vi "midi_TicsToTime.vi"(8 "error in (no error)":errorcluster, 9 "ticks per qnote":u16, 10 "tempo":u32[][](array[numeric]), 11 "notes in":u32[][](array[numeric])) -> (0 "error out":errorcluster, 2 "duration (s)":dbl, 3 "notes out":dbl[][](array[numeric]))   [LabVIEW 2013]
doc: "Convert the start times and durations from \"tics\" to seconds."
uses:
  <vilib>/Analysis/NI_AALPro.lvlib
panel:
  # "midi_TicsToTime"
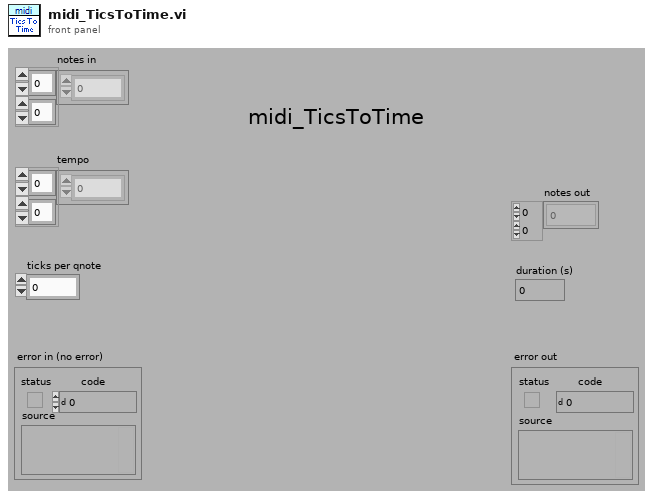
[diagram p1: front panel]
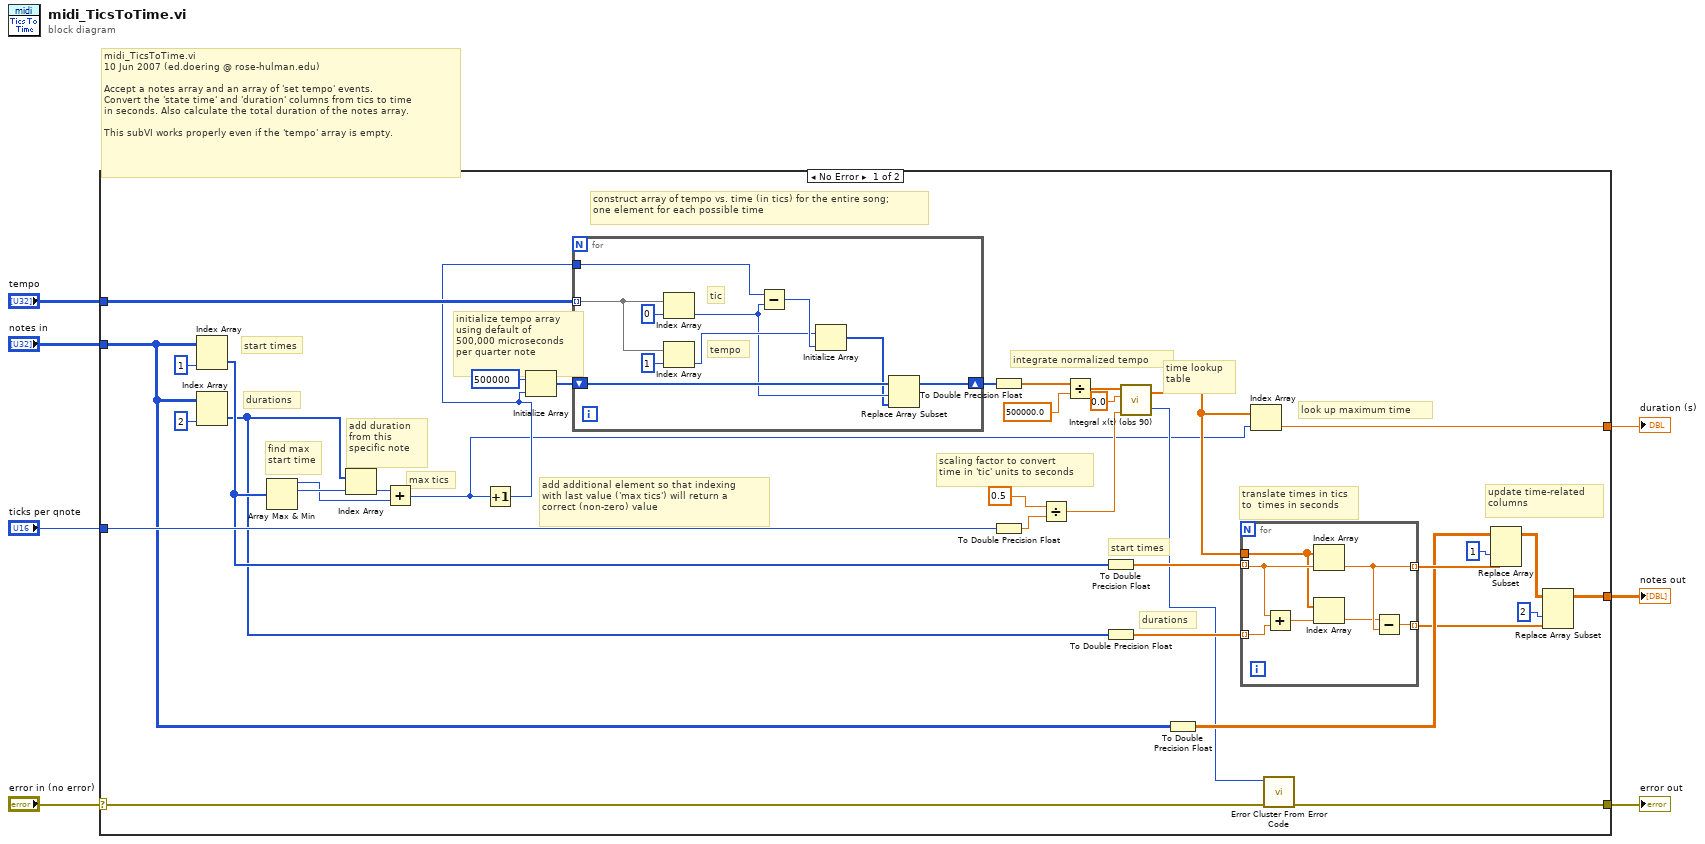
[diagram p0: block diagram]
diagram:
  # "midi_TicsToTime.vi\n10 Jun 2007 (ed.doering @ rose-hulman.edu)\n\nAccept a notes array and an array of 'set tempo' events.\nConvert the 'state time' and 'duration' columns from tics to time\nin seconds. Also calculate the total duration of the notes array.\n\nThis subVI works properly even if the 'tempo' array is empty."
  n1 = case shown="No Error" "error in (no error)" {
    selector: "error in (no error)" -> [w13 w61]
    tunnel: [w12 w61] -> w6
    tunnel: "tempo" -> [w36 _]
    tunnel: "notes in" -> [w18 _]
    tunnel: "ticks per qnote" -> [w27 _]
    tunnel: [w15 _] -> w2
    tunnel: [w8 _] -> w1
    frame No Error {
      # "add additional element so that indexing\nwith last value ('max tics') will return a\ncorrect (non-zero) value"
      # "look up maximum time"
      # "update time-related\ncolumns"
      # "translate times in tics\nto  times in seconds"
      # "durations"
      # "start times"
      # "time lookup\ntable"
      # "scaling factor to convert\ntime in 'tic' units to seconds"
      # "integrate normalized tempo"
      # "construct array of tempo vs. time (in tics) for the entire song;\none element for each possible time"
      # "initialize tempo array\nusing default of\n500,000 microseconds\nper quarter note"
      # "max tics"
      # "add duration \nfrom this\nspecific note"
      # "find max\nstart time"
      # "durations"
      # "start times"
      n2 = Index Array(array=w18, index (col)=1 ("disabled index (col)")) -> (element=w26:u32[])  [unwired: 1 in]
      n3 = Index Array(array=w18, index (col)=2 ("disabled index (col)")) -> (element=w25:u32[])  [unwired: 1 in]
      n4 = Array Max & Min(array=w26) -> (max value=w39:u32, max index (indices)=w41:i32)  [unwired: 2 out]
      n5 = Index Array(array=w25, index=w41) -> (element=w40:u32)
      n6 = Add(x=w40, y=w39) -> (x+y=w9:u32)
      n7 = Increment(x=w9) -> (x+1=w11:u32)
      n8 = Initialize Array(u32 500000 ("element"), w11) -> (w37:u32[])
      n9 = for {
        tunnel: w36 -> [w58] mode=indexing
        tunnel: w11 -> [w57]
        shift-right: [w51] -> w29
        shift-left: w37 -> [w54]
        # "tempo"
        # "tic"
        n10 = Index Array(array=w58, index=0) -> (element=w53:u32)
        n11 = Index Array(array=w58, index=1) -> (element=w55:u32)
        n12 = Subtract(x=w57, y=w53) -> (x-y=w56:u32)
        n13 = Initialize Array(w55, w56) -> (w52:u32[])
        n14 = Replace Array Subset(array=w54, new element=w52, index=w53) -> (w51:u32[])
      }
      n15 = To Double Precision Float(number=w29) -> (double precision float=w33:dbl[])
      n16 = To Double Precision Float(number=w27) -> (double precision float=w28:dbl)
      n17 = Divide(x=0.5, y=w28) -> (x/y=w30:dbl)
      n18 = Divide(x=w33, y=500000.0) -> (x/y=w32:dbl[])
      n19 = To Double Precision Float(number=w26) -> (double precision float=w24:dbl[])
      n20 = To Double Precision Float(number=w25) -> (double precision float=w23:dbl[])
      n21 = call <vilib>:"Integral x(t) (obs 90).vi"("dt"=w30, "initial condition"=0.0, "X"=w32) -> ("error"=w14:i32, "Integral X"=w10:dbl[])  [unwired: 1 in]
      n22 = To Double Precision Float(number=w18) -> (double precision float=w17:dbl[][])
      n23 = for {
        tunnel: w24 -> [w50] mode=indexing
        tunnel: w10 -> [w45]
        tunnel: [w47] -> w19 mode=indexing
        tunnel: w23 -> [w49] mode=indexing
        tunnel: [w44] -> w16 mode=indexing
        n24 = Add(x=w50, y=w49) -> (x+y=w48:dbl)
        n25 = Index Array(array=w45, index=w50) -> (element=w47:dbl)
        n26 = Index Array(array=w45, index=w48) -> (element=w46:dbl)
        n27 = Subtract(x=w46, y=w47) -> (x-y=w44:dbl)
      }
      n28 = Index Array(array=w10, index=w9) -> (element=w8:dbl)
      n29 = call <vilib>:"Error Cluster From Error Code.vi"("error in (no error)"=w13, "error code (0)"=w14) -> ("error out"=w12:errorcluster)  [unwired: 7 in]
      n30 = Replace Array Subset(array=w17, new element=w19, index (col)=1 ("disabled index (col)")) -> (w20:dbl[][])  [unwired: 1 in]
      n31 = Replace Array Subset(array=w20, new element=w16, index (col)=2 ("disabled index (col)")) -> (w15:dbl[][])  [unwired: 1 in]
    }
    frame Error {
    }
  }
  "error out" <- w6
  "notes out" <- w2
  "duration (s)" <- w1
